vi "Z6_Beamline_Chief.contents.vi"   [LabVIEW 2014, in "Z6_Beamline_Chief.lvlib"]
doc: "This class is forseen to inspect the PHELIX beamline and to select the mode. Additional several settings can be chosen.\n\nThis class is part of the PHELIX user layer."
uses:
  Z6_Beamline_Chief.lvlib
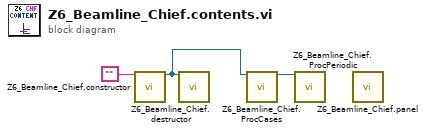
[diagram p0: block diagram]
diagram:
  n1 = call "Z6_Beamline_Chief.constructor.vi"("name"="") -> ("i ref out"=w1:refnum<vi>)  [unwired: 16 in, 2 out]
  n2 = call "Z6_Beamline_Chief.destructor.vi"("i ref in"=w1) -> ()  [unwired: 18 in, 1 out]
  n3 = call "Z6_Beamline_Chief.ProcCases.vi"("i ref in"=w1) -> ("i ref out"=w2:refnum<vi>)  [unwired: 16 in, 2 out]
  n4 = call "Z6_Beamline_Chief.ProcPeriodic.vi"("i ref in"=w2) -> ()  [unwired: 16 in, 3 out]
  n5 = call "Z6_Beamline_Chief.panel.vi"() -> ()  [unwired: 19 in, 1 out]
